vi "Write CSGL.vi"(8 "error in (no error)":errorcluster, 9 "Numeric":csg, 10 "Tag":string, 11 "Omni_Bus in":refnum<class "Omni_Bus.lvclass">) -> (0 "error out":errorcluster, 3 "Omni_Bus out":refnum<class "Omni_Bus.lvclass">)   [LabVIEW 2021, in "Omni_Bus.lvclass"]
uses:
  Omni_Bus.lvclass
  <vilib>/TSA/Abstract Data Classes/Abs_Types/Complex Single Float/Abs_Complex Single Float.lvclass
  C:/Program Files (x86)/National Instruments/LabVIEW 2021/vi.lib/TSA/Abstract Data Classes/Abs_Types/Type/Abs_Type.lvclass
  Omni_Bus.lvclass/Omni_Bus.ctl
  C:/Program Files (x86)/National Instruments/LabVIEW 2021/vi.lib/TSA/Abstract Data Classes/Abs_Types/Floating Point/Abs_Floating Point.lvclass
  C:/Program Files (x86)/National Instruments/LabVIEW 2021/vi.lib/TSA/Abstract Data Classes/Abs_Types/Numeric/Abs_Numeric.lvclass
  C:/Program Files (x86)/National Instruments/LabVIEW 2021/vi.lib/TSA/Abstract Data Classes/Abs_Types/Value/Abs_Value.lvclass
  C:/Program Files (x86)/National Instruments/LabVIEW 2021/vi.lib/TSA/Abstract Data Classes/Abs_Types/Complex Single Float/Abs_Complex Single Float.lvclass
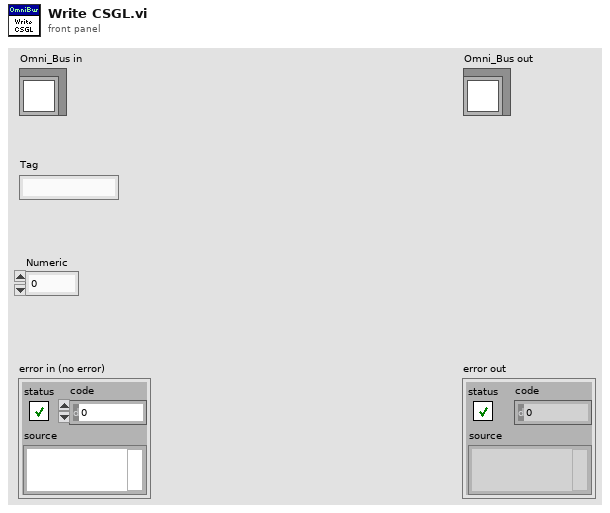
[diagram p1: front panel]
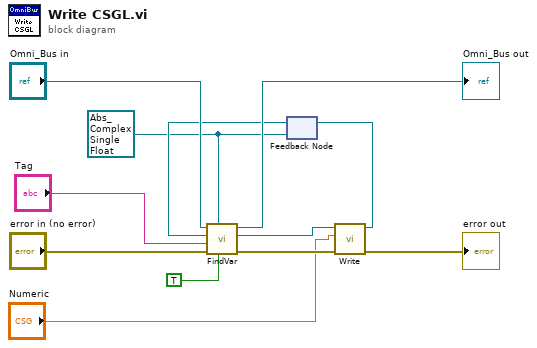
[diagram p0: block diagram]
diagram:
  w1 = refnum<class "Abs_Complex Single Float.lvclass"> refnum ("Double Float.lvclass_340760 out")
  n1 = feedback #1(w1) -> (w4:refnum<class "Abs_Complex Single Float.lvclass">)
  n2 = call "FindVar.vi"("Write?"=TRUE, "Abs_Type"=w1, "error in (no error)"="error in (no error)", "Tag"="Tag", "Abs_Type Default"=w4, "Var Bus in"="Omni_Bus in") -> ("error out"=w8:errorcluster, "Abs_Type Found"=w5:refnum<class "Abs_Complex Single Float.lvclass">, "Var Bus out"=→"Omni_Bus out":refnum<class "Omni_Bus.lvclass">)  [unwired: 2 in, 1 out]
  n3 = call-dynamic "Write.vi"("error in (no error)"=w8, "Value"="Numeric", "Double Float.lvclass_340760 in"=w5) -> ("error out"=→"error out":errorcluster, "Double Float.lvclass_340760 out"=w6:refnum<class "Abs_Complex Single Float.lvclass">)  [unwired: 7 in]
  n4 = feedback-in #1(w6) -> ()
